vi "Agilent VNA Read Power.vi"(6 "Channel":i8=1 min=1 max=99 step=1, 7 "Agilent VNA":T1, 8 "error in (no error)":errorcluster, 11 "VISA Resource Name":refnum<visa-resource-name>) -> (0 "error out":errorcluster, 1 "Source Power Min, dBm":dbl, 2 "Source Power, dBm":dbl, 3 "dup VISA Resource Name":refnum<visa-resource-name>, 5 "Source Power Max, dBm":dbl)   [LabVIEW 2011]
doc: "This vi sets the power range. Only works on the HP 8753D."
uses:
  TypeDefs/Agilent VNA Instrument Info.ctl
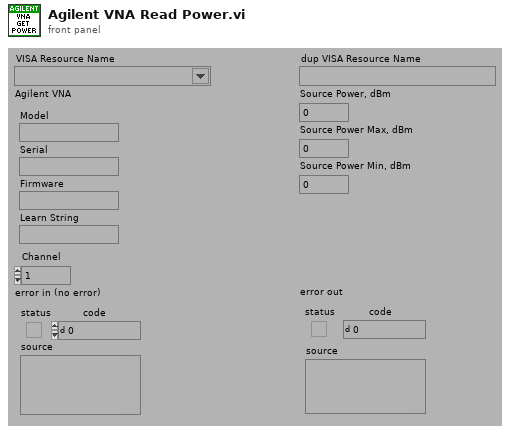
[diagram p1: front panel]
types:
  T1 = typedef "Agilent VNA Instrument Info.ctl" = cluster{"Model":string, "Serial":string, "Firmware":string, "Learn String":string}
  T2 = typedef "Agilent VNA Model.ctl" = enum16{"Not Supported", "8510X", "8719X", "8720X", "8722X", "8753X", "ENA", "PNA", "Field Fox"}
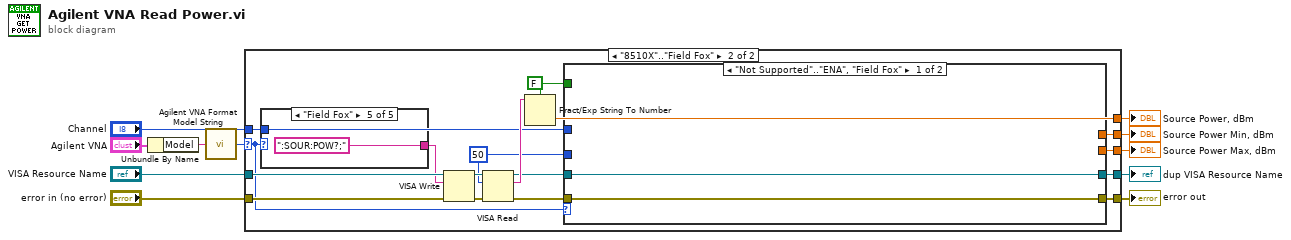
[diagram p0: block diagram]
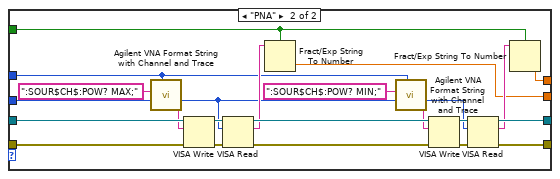
[diagram p3: hidden frame]
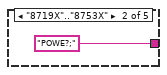
[diagram p5: hidden frame]
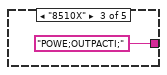
[diagram p6: hidden frame]
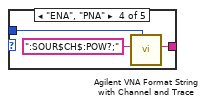
[diagram p7: hidden frame]
diagram:
  n1 = Unbundle By Name("Agilent VNA") -> ("Model"=w2:string)
  n2 = call "Agilent VNA Format Model String.vi"("Model"=w2) -> ("Model"=w1:T2)
  n3 = case shown="\"8510X\"..\"Field Fox\"" w1 {
    selector: w1 -> [_ w14]
    tunnel: "VISA Resource Name" -> [w13 w30]
    tunnel: "error in (no error)" -> [w12 w29]
    tunnel: [_ w24] -> w9
    tunnel: [w13 w21] -> w8
    tunnel: [w12 w20] -> w7
    tunnel: "Channel" -> [_ w17]
    tunnel: [_ w16] -> w5
    tunnel: [_ w15] -> w4
    frame "Not Supported" {
    }
    frame "8510X".."Field Fox" {
      w19 = FALSE ("use system decimal point (T)")
      w18 = u32 50 ("byte count")
      n4 = case shown="\"Field Fox\"" w14 {
        tunnel: [_ "POWE?;" "POWE;OUTPACTI;" w57 ":SOUR:POW?;"] -> w26
        tunnel: w17 -> [_ _ _ w56 _]
        frame "Not Supported" {
        }
        frame "8719X".."8753X" {
        }
        frame "8510X" {
        }
        frame "ENA", "PNA" {
          n5 = call "Agilent VNA Format String with Channel and Trace.vi"("Channel"=w56, "String"=":SOUR$CH$:POW?;") -> ("String Out"=w57:string)  [unwired: 1 in, 6 out]
        }
        frame "Field Fox" {
        }
      }
      n6 = VISA Write(VISA resource name=w30, write buffer=w26, error in (no error)=w29) -> (VISA resource name out=w28:refnum<visa-resource-name>, error out=w27:errorcluster)  [unwired: 1 out]
      n7 = VISA Read(VISA resource name=w28, byte count=w18, error in (no error)=w27) -> (VISA resource name out=w23:refnum<visa-resource-name>, read buffer=w25:string, error out=w22:errorcluster)  [unwired: 1 out]
      n8 = Fract/Exp String To Number(use system decimal point (T)=w19, string=w25) -> (number=w24:dbl)  [unwired: 3 out]
      n9 = case shown="\"Not Supported\"..\"ENA\", \"Field Fox\"" w14 {
        tunnel: w23 -> [w31 w49]
        tunnel: w22 -> [w32 w48]
        tunnel: [w31 w45] -> w21
        tunnel: [w32 w44] -> w20
        tunnel: w19 -> [_ w40]
        tunnel: w18 -> [_ w42]
        tunnel: w17 -> [_ w33]
        tunnel: [_ w35] -> w16
        tunnel: [_ w34] -> w15
        frame "Not Supported".."ENA", "Field Fox" {
        }
        frame "PNA" {
          n10 = call "Agilent VNA Format String with Channel and Trace.vi"("Channel"=w33, "String"=":SOUR$CH$:POW? MAX;") -> ("String Out"=w38:string)  [unwired: 1 in, 6 out]
          n11 = VISA Write(VISA resource name=w49, write buffer=w38, error in (no error)=w48) -> (VISA resource name out=w52:refnum<visa-resource-name>, error out=w53:errorcluster)  [unwired: 1 out]
          n12 = VISA Read(VISA resource name=w52, byte count=w42, error in (no error)=w53) -> (VISA resource name out=w46:refnum<visa-resource-name>, read buffer=w43:string, error out=w47:errorcluster)  [unwired: 1 out]
          n13 = Fract/Exp String To Number(use system decimal point (T)=w40, string=w43) -> (number=w34:dbl)  [unwired: 3 out]
          n14 = call "Agilent VNA Format String with Channel and Trace.vi"("Channel"=w33, "String"=":SOUR$CH$:POW? MIN;") -> ("String Out"=w36:string)  [unwired: 1 in, 6 out]
          n15 = VISA Write(VISA resource name=w46, write buffer=w36, error in (no error)=w47) -> (VISA resource name out=w51:refnum<visa-resource-name>, error out=w50:errorcluster)  [unwired: 1 out]
          n16 = VISA Read(VISA resource name=w51, byte count=w42, error in (no error)=w50) -> (VISA resource name out=w45:refnum<visa-resource-name>, read buffer=w41:string, error out=w44:errorcluster)  [unwired: 1 out]
          n17 = Fract/Exp String To Number(use system decimal point (T)=w40, string=w41) -> (number=w35:dbl)  [unwired: 3 out]
        }
      }
    }
  }
  "dup VISA Resource Name" <- w8
  "error out" <- w7
  "Source Power, dBm" <- w9
  "Source Power Min, dBm" <- w5
  "Source Power Max, dBm" <- w4
